vi "test dot display.vi"() -> ()   [LabVIEW 2016]
uses:
  <vilib>/Utility/miscctls.llb/LVRectTypeDef.ctl
  <vilib>/Utility/miscctls.llb/LVBoundsTypeDef.ctl
  <vilib>/Utility/miscctls.llb/LVPositionTypeDef.ctl
  <vilib>/Analysis/baseanly.llb/Mean (DBL).vi
  <vilib>/Analysis/NI_AALBase.lvlib
panel:
  out "x/y":dbl
  out "Array 4":dbl[](array[numeric])
  in  "Button Size 2":T1
  out "Array 3":dbl[](array[numeric])
  out "Front Panel Window:Window Bounds":T2
  out "error out 2":errorcluster
  out "Array 2":i32[](array[numeric])
  out "Array":string[](array[string])
  out "cycle results dbl":dbl[][](array[numeric])
  out "Time":u32
  out "error out":errorcluster
  out "cycle value 40":bool
  out "cycle value 39":bool
  out "cycle value 38":bool
  out "cycle value 37":bool
  out "cycle value 36":bool
  out "cycle value 35":bool
  out "cycle value 34":bool
  out "cycle value 33":bool
  out "cycle value 32":bool
  out "cycle value 31":bool
  out "cycle value 30":bool
  out "cycle value 29":bool
  out "cycle value 28":bool
  out "cycle value 27":bool
  out "cycle value 26":bool
  out "cycle value 25":bool
  out "cycle value 24":bool
  out "cycle value 23":bool
  out "cycle value 22":bool
  out "cycle value 21":bool
  out "cycle value 20":bool
  out "cycle value 19":bool
  out "cycle value 18":bool
  out "cycle value 17":bool
  out "cycle value 16":bool
  out "cycle value 15":bool
  out "cycle value 14":bool
  out "cycle value 13":bool
  out "cycle value 12":bool
  out "cycle value 11":bool
  out "cycle value 10":bool
  out "cycle value 9":bool
  out "cycle value 8":bool
  out "cycle value 7":bool
  out "cycle value 6":bool
  out "cycle value 5":bool
  out "cycle value 4":bool
  out "cycle value 3":bool
  out "cycle value 2":bool
  out "cycle value":bool
  out "sequence result 10":bool
  out "sequence result 9":bool
  out "sequence result 8":bool
  out "sequence result 7":bool
  out "sequence result 6":bool
  out "sequence result 5":bool
  out "sequence result 4":bool
  out "sequence result 3":bool
  out "sequence result 2":bool
  out "sequence result":bool
  out "sample result":bool
  in  "stop":bool
types:
  T1 = typedef "LVBoundsTypeDef.ctl" = cluster{"Width":u32, "Height":u32}
  T2 = typedef "LVRectTypeDef.ctl" = cluster{"Left":i16, "Top":i16, "Right":i16, "Bottom":i16}
  T3 = enum8{"Enabled", "Disabled", "Disabled and Grayed Out"}
  T4 = typedef "LVPositionTypeDef.ctl" = cluster{"Left":i32, "Top":i32}
  T5 = typedef "cycle results control.ctl" = cluster{"sample info":string[][], "cycle results labels":string[], "cycle results dbl":dbl[][]}
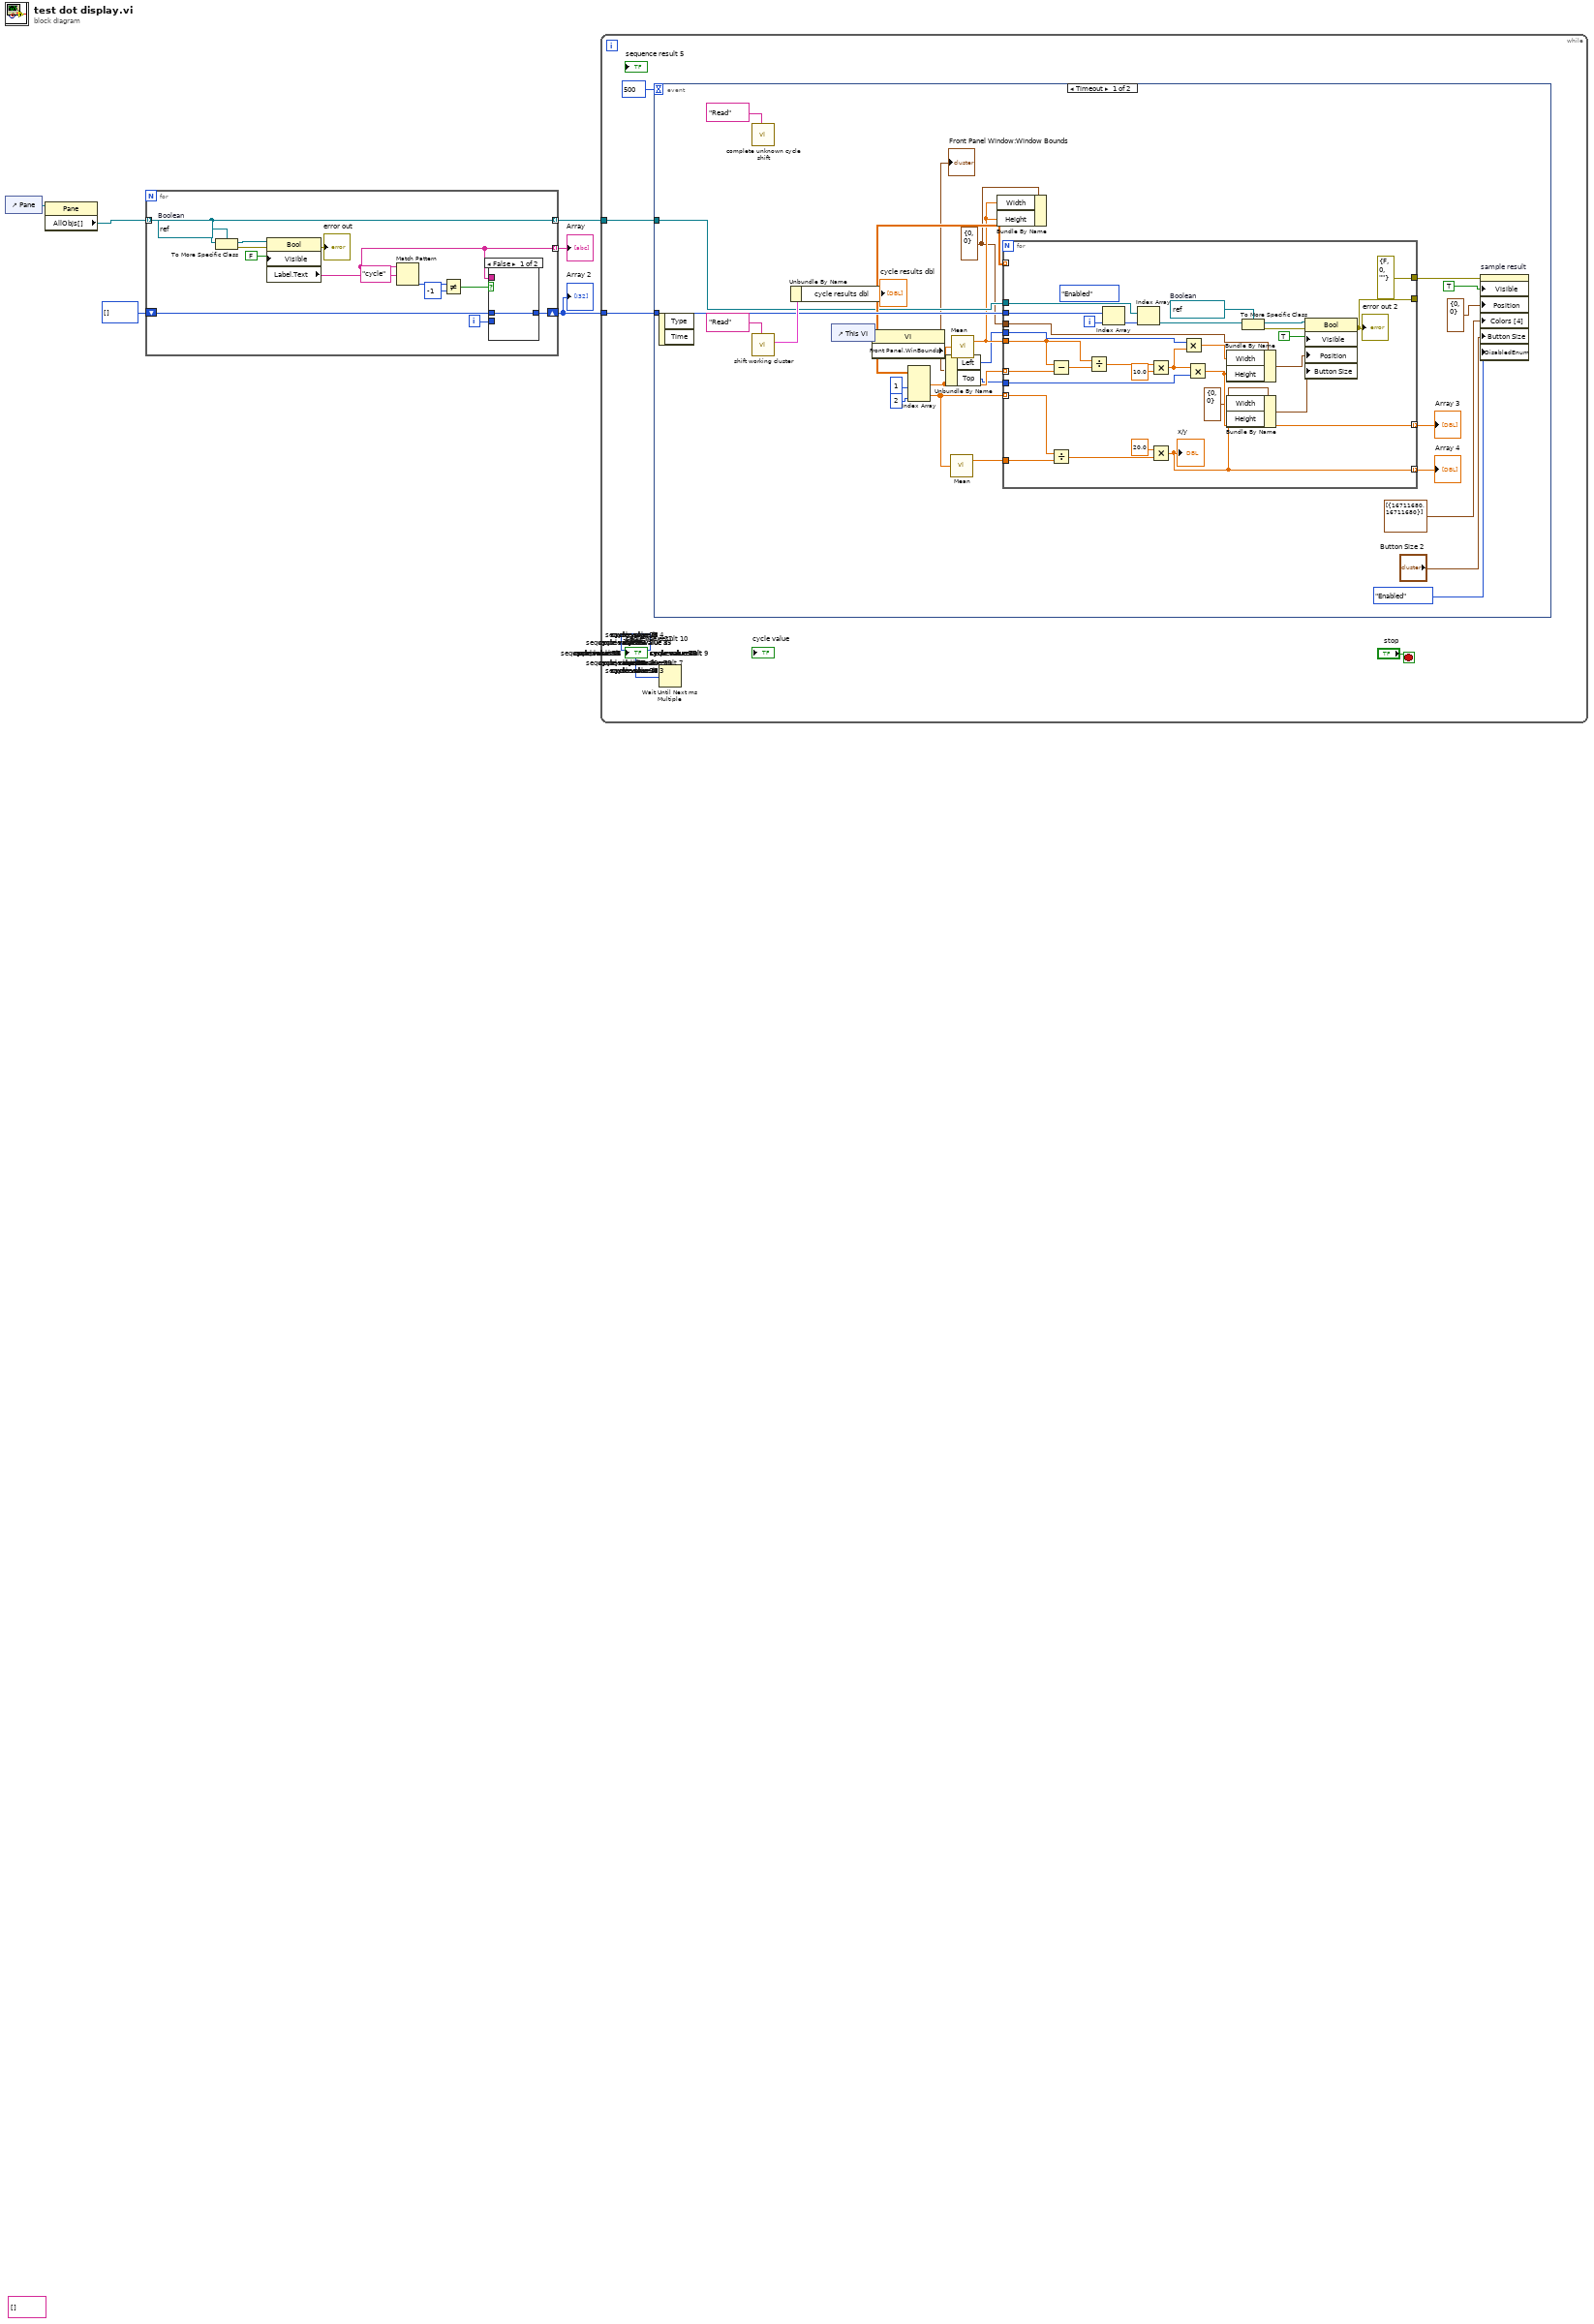
[diagram p0: block diagram]
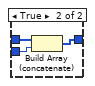
[diagram p2: hidden frame]
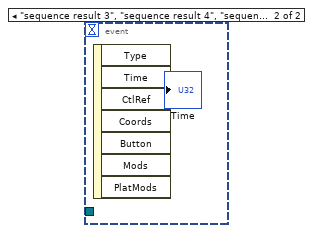
[diagram p3: hidden frame]
diagram:
  (unwired) string[] []
  n1 = control-ref of="Pane"() -> (w5:refnum<vi>)
  n2 = property class="Pane"(reference=w5) -> ("AllObjs[]"=w6:refnum<vi>[])  [unwired: 1 in, 2 out]
  n3 = for {
    tunnel: w6 -> [w19] mode=indexing
    tunnel: [w19] -> w4 mode=indexing
    tunnel: [w10] -> w3 mode=indexing
    shift-right: [w7] -> w1
    shift-left: i32[] [] -> [w9]
    i -> [w8]
    w20 = refnum<vi> refnum  # Boolean
    n4 = To More Specific Class(target class=w20, reference=w19) -> (specific class reference=w18:refnum<vi>, error out=w15:errorcluster)  [unwired: 1 in]
    n5 = property class="Bool"(reference=w18, error in=w15, "Visible"=FALSE) -> (error out=→"error out":errorcluster, "Label.Text"=w10:string)  [unwired: 1 out]
    n6 = Match Pattern(string=w10, regular expression="cycle") -> (offset past match=w13:i32)  [unwired: 1 in, 3 out]
    n7 = Not Equal?(x=w13, y=-1) -> (x != y?=w11:bool)
    n8 = case shown="False" w11 {
      tunnel: w10 -> [_ _]
      tunnel: w9 -> [w21 w24]
      tunnel: w8 -> [_ w23]
      tunnel: [w21 w22] -> w7
      frame False {
      }
      frame True {
        n9 = Build Array (concatenate)(w24, w23) -> (w22:i32[])
      }
    }
  }
  "Array" <- w3
  "Array 2" <- w1
  n10 = while {
    tunnel: w4 -> [w26]
    tunnel: w1 -> [w25]
    stop <- "stop" stop-if-true
    n11 = event shown="[0] Timeout" {
      selector: _ -> [_ _]
      dyn-events: _ -> [_ _]
      timeout: 500 -> [_ _]
      tunnel: w26 -> [w48 _]
      tunnel: w25 -> [w51 _]
      event Timeout {
        w34 = T1 {"Width"=0, "Height"=0} ("Bounds")
        n12 = event-data() -> ()  [unwired: 1 in, 2 out]
        n13 = call "complete unknown cycle shift.vi"("read write shift"="Read") -> ()  [unwired: 9 in, 2 out]
        n14 = call "shift working cluster.vi"("read write shift"="Read") -> ("cycle results cluster out"=w52:T5)  [unwired: 9 in, 1 out]
        n15 = Unbundle By Name(w52) -> ("cycle results dbl"=w50:dbl[][])
        "cycle results dbl" <- w50
        n16 = control-ref of="This VI"() -> (w41:refnum<vi>)
        n17 = property class="VI"(reference=w41) -> ("Front Panel.WinBounds"=w40:T2)  [unwired: 1 in, 2 out]
        "Front Panel Window:Window Bounds" <- w40
        n18 = Index Array(array=w50, index (col) #1=1 ("disabled index (col)"), index (col) #2=2 ("index (col)")) -> (element #1=w47:dbl[], element #2=w33:dbl[])  [unwired: 2 in]
        n19 = Unbundle By Name(w40) -> ("Left"=w39:i16, "Top"=w38:i16)
        n20 = call-poly <vilib>:"Mean.vi"("X"=w33) -> ("mean"=w31:dbl)  [unwired: 1 out]
        n21 = call-poly <vilib>:"Mean.vi"("X"=w47) -> ("mean"=w42:dbl)  [unwired: 1 out]
        n22 = Bundle By Name(cluster=w34, "Width"=w42, "Height"=w42) -> ()  [unwired: 1 out]
        n23 = for {
          tunnel: w50 -> [_] mode=indexing
          tunnel: w51 -> [w84]
          tunnel: w48 -> [w81]
          tunnel: w34 -> [w76]
          tunnel: w47 -> [w71] mode=indexing
          tunnel: [w73] -> _
          tunnel: [errorcluster {"status"=FALSE, "code"=0, "source"=""} ("error out 3")] -> w43
          tunnel: w42 -> [w70]
          tunnel: w39 -> [w68]
          tunnel: w38 -> [w67]
          tunnel: [w65] -> w37 mode=indexing
          tunnel: w31 -> [w61]
          tunnel: w33 -> [w60] mode=indexing
          tunnel: [w55] -> w32 mode=indexing
          i -> [w83]
          (unwired) T3."Enabled" ("Disabled")
          w80 = refnum<vi> refnum  # Boolean
          n24 = Subtract(x=w70, y=w71) -> (x-y=w69:dbl)
          n25 = Divide(x=w60, y=w61) -> (x/y=w57:dbl)
          n26 = Divide(x=w70, y=w69) -> (x/y=w64:dbl)
          n27 = Index Array(array=w84, index=w83) -> (element=w82:i32)
          n28 = Index Array(array=w81, index=w82) -> (element=w79:refnum<vi>)
          n29 = Multiply(x=w64, y=10.0) -> (x*y=w62:dbl)
          n30 = Multiply(x=20.0, y=w57) -> (x*y=w55:dbl)
          "x/y" <- w55
          n31 = Multiply(x=w68, y=w62) -> (x*y=w66:dbl)
          n32 = Multiply(x=w62, y=w67) -> (x*y=w65:dbl)
          n33 = Bundle By Name(cluster=w76, "Width"=w66, "Height"=w65) -> (w75:T1)
          n34 = Bundle By Name(cluster=T1 {"Width"=0, "Height"=0} ("Button Size"), "Width"=w55, "Height"=w55) -> (w58:T1)
          n35 = To More Specific Class(target class=w80, reference=w79) -> (specific class reference=w78:refnum<vi>, error out=w74:errorcluster)  [unwired: 1 in]
          n36 = property class="Bool"(reference=w78, error in=w74, "Visible"=TRUE, "Position"=w75, "Button Size"=w58) -> (error out=w73:errorcluster)  [unwired: 1 out]
          "error out 2" <- w73
        }
        "Array 3" <- w37
        "Array 4" <- w32
        n37 = property on="sample result" class="Bool (strict)"(error in=w43, "Visible"=TRUE, "Position"=T4 {"Left"=0, "Top"=0}, "Colors [4]"=cluster{u32, u32}[] [{16711680, 16711680}], "Button Size"="Button Size 2", "DisabledEnum"=T3."Enabled" ("Disabled")) -> ()  [unwired: 1 in, 2 out]
      }
      event "sequence result 3", "sequence result 4", "sequence result 5", "sequence result 6", "sequence result 7", "sequence result 8", "sequence result 9", "sequence result 10", "cycle value", "cycle value 2", "cycle value 3", "cycle value 4", "cycle value 5", "cycle value 6", "sample result": Mouse Down {
        n38 = event-data() -> ("Time"=→"Time":u32)  [unwired: 1 in, 6 out]
      }
    }
    n39 = Wait Until Next ms Multiple(millisecond multiple=u32 1000) -> ()  [unwired: 1 out]
  }
